vi "Update Buttons.vi"(8 "error in":errorcluster, 11 "Button Manager in":refnum<class "Button Manager.lvclass">) -> (0 "error out":errorcluster, 3 "Button Manager out":refnum<class "Button Manager.lvclass">)   [LabVIEW 2020, in "Navigation.lvlib" / "Button Manager.lvclass"]
doc: "____\nHAMPEL SOFTWARE ENGINEERING v2.6.0 (2023-12-19 10:54)"
uses:
  Button Manager.lvclass
  Button Manager.lvclass/Button Manager.ctl
  Button Def.ctl
  Top Control.ctl
  Sub Control.ctl
  <vilib>/Utility/error.llb/Error Cluster From Error Code.vi
  <vilib>/ErrorRing/Error Ring.xnode
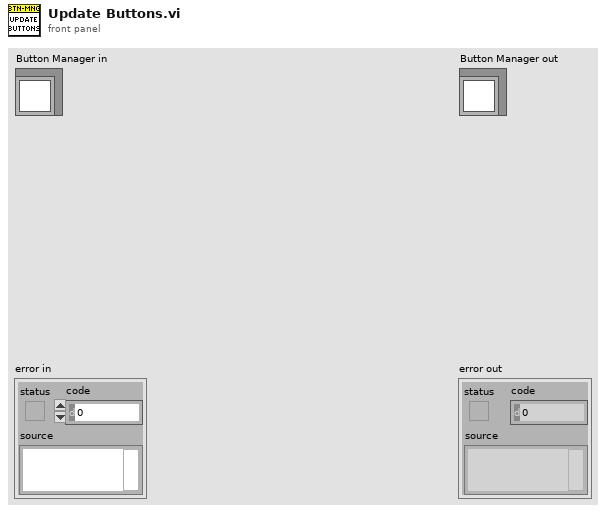
[diagram p1: front panel]
types:
  T1 = typedef "Navigation.lvlib/Button Manager.lvclass/Button Def.ctl" = cluster{"Top-Ctl Ref":refnum<vi>, "Sub-Ctl Ref":refnum<vi>, "Button Object":T2}
  T2 = typedef "Navigation.lvlib/Button Manager.lvclass/Top Control.ctl" = cluster{"name":string, "caption":string, "tooltip":string, "enabled_state":string, "action":string, "display_scenario":string, "sub":T3[]}
  T3 = typedef "Navigation.lvlib/Button Manager.lvclass/Sub Control.ctl" = cluster{"name":string, "tooltip":string, "enabled_state":string, "content":string[], "retain value":bool}
  T4 = enum8{"Enabled", "Disabled", "Disabled and Grayed Out"}
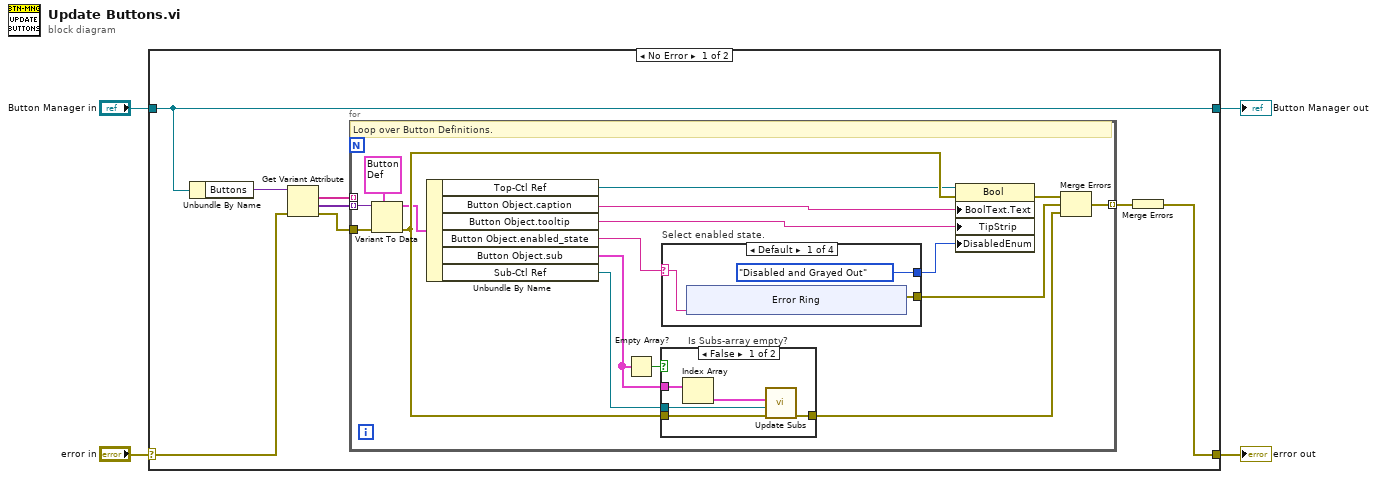
[diagram p0: block diagram]
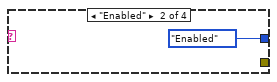
[diagram p3: hidden frame]
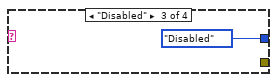
[diagram p4: hidden frame]
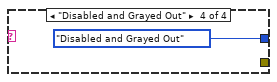
[diagram p5: hidden frame]
diagram:
  n1 = case shown="No Error" "error in" {
    selector: "error in" -> [w10 w50]
    tunnel: [w5 w50] -> w3
    tunnel: [w12 w49] -> w1
    tunnel: "Button Manager in" -> [w12 w49]
    frame No Error {
      n2 = Unbundle By Name(w12) -> ("Buttons"=w11:variant)
      n3 = Get Variant Attribute(Variant=w11, error in=w10) -> (names=w9:string[], values=w8:variant[], error out=w7:errorcluster)  [unwired: 2 in, 1 out]
      n4 = for {
        tunnel: w9 -> [_] mode=indexing
        tunnel: w8 -> [w27] mode=indexing
        tunnel: w7 -> [w26]
        tunnel: [w22] -> w6 mode=indexing
        # "Loop over Button Definitions."
        n5 = Variant To Data(error in=w26, type=T1 {"Top-Ctl Ref"=refnum, "Sub-Ctl Ref"=refnum, "Button Object"={"name"="", "caption"="", "tooltip"="", "enabled_state"="", "action"="", "display_scenario"="", "sub"=[]}} ("Button Def"), Variant=w27) -> (data=w25:T1, error out=w29:errorcluster)
        n6 = Unbundle By Name(w25) -> ("Top-Ctl Ref"=w17:refnum<vi>, "Button Object.caption"=w20:string, "Button Object.tooltip"=w19:string, "Button Object.enabled_state"=w18:string, "Button Object.sub"=w15:T3[], "Sub-Ctl Ref"=w14:refnum<vi>)
        n7 = Empty Array?(array=w15) -> (empty?=w16:bool)
        n8 = case "Is Subs-array empty?" shown="False" w16 {
          tunnel: w15 -> [w34 _]
          tunnel: w14 -> [w32 _]
          tunnel: w29 -> [w31 w35]
          tunnel: [w30 w35] -> w13
          frame False {
            n9 = Index Array(array=w34) -> (element=w33:T3)  [unwired: 1 in]
            n10 = call "Update Subs.vi"("error in"=w31, "Sub-Ctl Ref"=w32, "Sub Control"=w33) -> ("error out"=w30:errorcluster)  [unwired: 8 in]
          }
          frame True {
          }
        }
        n11 = case "Select enabled state." shown="Default" w18 {
          selector: w18 -> [w37 _ _ _]
          tunnel: [T4."Disabled and Grayed Out" ("Disabled") T4."Enabled" ("Disabled") T4."Disabled" ("Disabled") T4."Disabled and Grayed Out" ("Disabled")] -> w23
          tunnel: [w36 _ _ _] -> w21
          frame Default {
            n12 = xnode "Error Ring"("parameter 0"=w37) -> ("error out"=w36:errorcluster)
          }
          frame "Enabled" {
          }
          frame "Disabled" {
          }
          frame "Disabled and Grayed Out" {
          }
        }
        n13 = property class="Bool"(reference=w17, error in=w29, "BoolText.Text"=w20, "TipStrip"=w19, "DisabledEnum"=w23) -> (error out=w24:errorcluster)  [unwired: 1 out]
        n14 = Merge Errors(w24, w21, w13) -> (w22:errorcluster)
      }
      n15 = Merge Errors(w6) -> (w5:errorcluster)
    }
    frame Error {
    }
  }
  "error out" <- w3
  "Button Manager out" <- w1
